vi "output csv buffer overflow.vi"(8 "error in (no error)":errorcluster caption="エラー入力（エラーなし）", 9 "ファイルパス (ダイアログを使用)":path, 10 "buffer remains":u32[][](array[numeric]), 11 "time":dbl[](array[numeric])) -> (0 "error out":errorcluster caption="エラー出力", 3 "path":path)   [LabVIEW 2018]
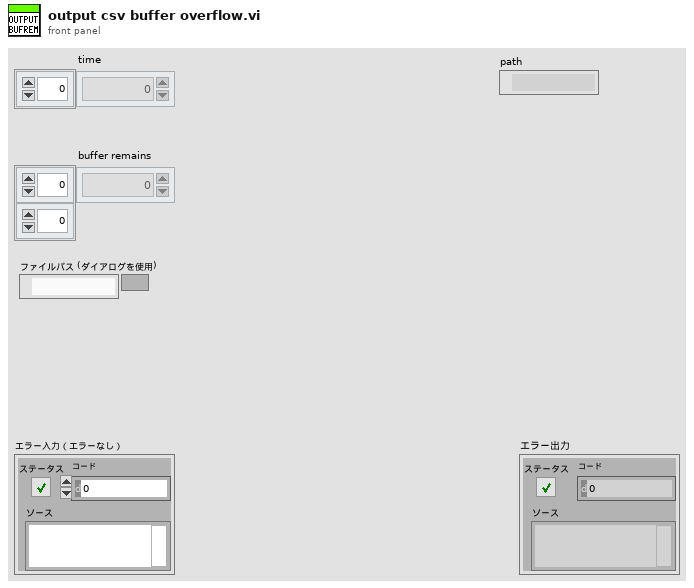
[diagram p1: front panel]
types:
  T1 = enum16{"open", "replace", "create", "open or create", "replace or create", "replace or create with confirmation"}
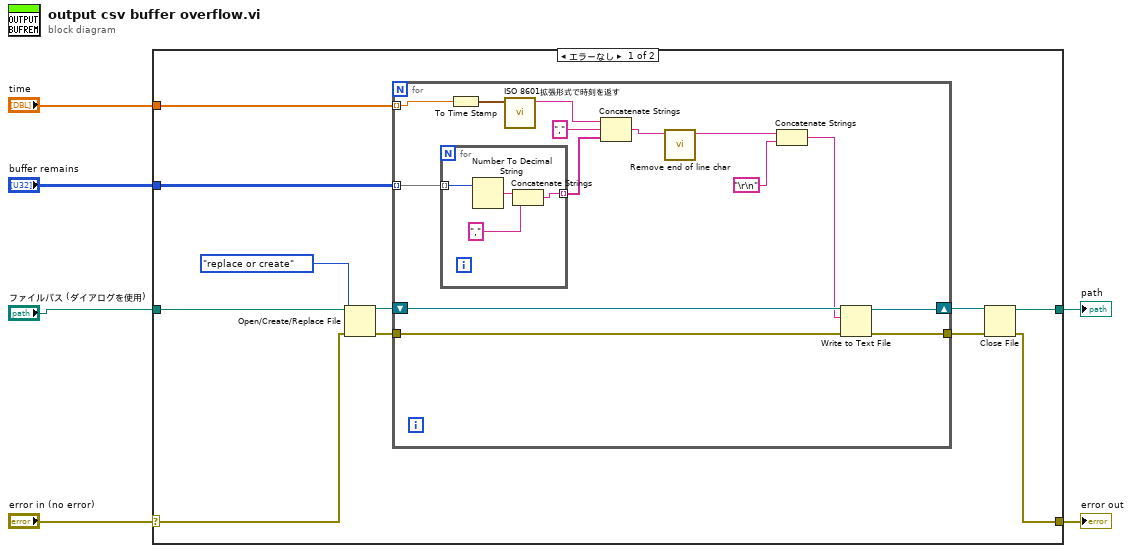
[diagram p0: block diagram]
diagram:
  n1 = case shown="エラーなし" "error in (no error)" {
    selector: "error in (no error)" -> [w7 w36]
    tunnel: [w12 w36] -> w5
    tunnel: "buffer remains" -> [w10 _]
    tunnel: [w11 _] -> w3
    tunnel: "time" -> [w9 _]
    tunnel: "ファイルパス (ダイアログを使用)" -> [w8 _]
    frame No Error {
      n2 = Open/Create/Replace File(file path (use dialog)=w8, error in=w7, operation (0:open)=T1."replace or create" ("操作 (0:open)")) -> (refnum out=w15:refnum<file>, error out=w14:errorcluster)  [unwired: 3 in, 1 out]
      n3 = for {
        shift-right: [w31] -> w16
        shift-left: w15 -> [w30]
        tunnel: w14 -> [w29]
        tunnel: w10 -> [w23] mode=indexing
        tunnel: [w28] -> w13
        tunnel: w9 -> [w20] mode=indexing
        n4 = for {
          tunnel: w23 -> [w35] mode=indexing
          tunnel: [w33] -> w27 mode=indexing
          n5 = Number To Decimal String(number=w35) -> (decimal integer string=w34:string)  [unwired: 1 in]
          n6 = Concatenate Strings(w34, "," ("文字列")) -> (w33:string)
        }
        n7 = To Time Stamp(1:w20) -> (0:w19:timestamp)
        n8 = call "ISO 8601拡張形式で時刻を返す.vi"("タイムスタンプ"=w19) -> ("日付/時間文字列"=w18:string)  [unwired: 9 in, 1 out]
        n9 = Concatenate Strings(w18, "," ("文字列"), w27) -> (w22:string)
        n10 = call "Remove end of line char.vi"("文字列"=w22) -> ("文字列 out"=w21:string)  [unwired: 9 in, 1 out]
        n11 = Concatenate Strings(w21, "\r\n") -> (w25:string)
        n12 = Write to Text File(file (use dialog)=w30, text=w25, error in=w29) -> (refnum out=w31:refnum<file>, error out=w28:errorcluster)  [unwired: 1 in, 1 out]
      }
      n13 = Close File(refnum=w16, error in=w13) -> (path=w11:path, error out=w12:errorcluster)
    }
    frame Error {
    }
  }
  "error out" <- w5
  "path" <- w3
